vi "createState.vi"(8 "error in (no error)":errorcluster, 10 "State:":T1, 11 "StateFactory in":refnum<class "StateFactory.lvclass">) -> (0 "error out":errorcluster, 2 "State.lvclass":refnum<class "State.lvclass">, 3 "StateFactory out":refnum<class "StateFactory.lvclass">)   [LabVIEW 2013, in "StateFactory.lvclass"]
uses:
  StateFactory.lvclass
  Typedefs/StateSelector.ctl
  State/State.lvclass
  States/DataOnDemandState/DataOnDemandState.lvclass
  States/DataStreamingState/DataStreamingState.lvclass
  States/FaultState/FaultState.lvclass
  States/OffState/OffState.lvclass
  States/StandbyState/StandbyState.lvclass
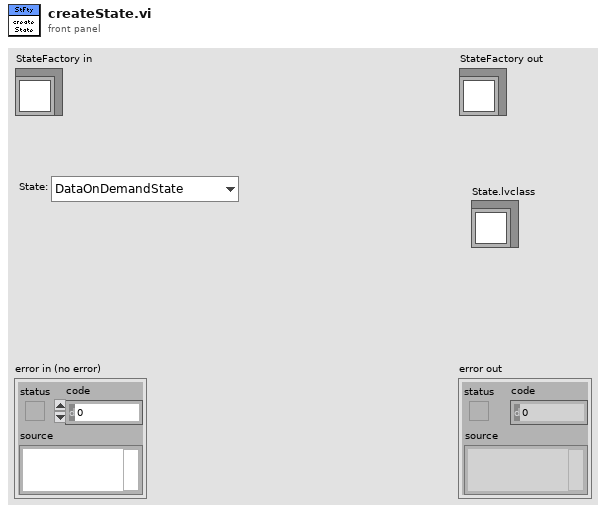
[diagram p1: front panel]
types:
  T1 = typedef "StateSelector.ctl" = enum16{"DataOnDemandState", "DataStreamingState", "FaultState", "OffState", "StandbyState"}
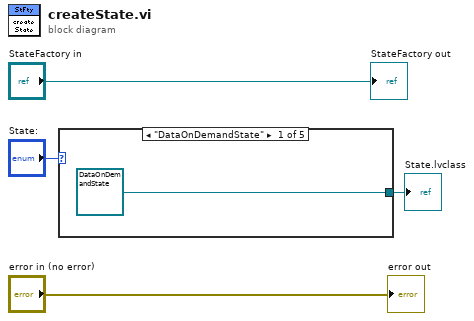
[diagram p0: block diagram]
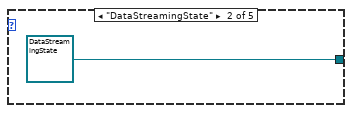
[diagram p2: hidden frame]
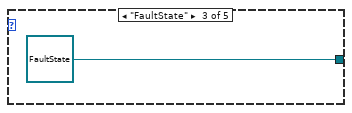
[diagram p3: hidden frame]
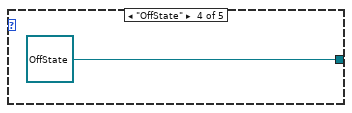
[diagram p4: hidden frame]
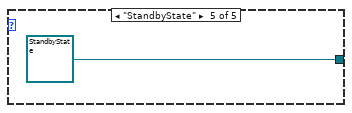
[diagram p5: hidden frame]
diagram:
  n1 = case shown="\"DataOnDemandState\"" "State:" {
    tunnel: [refnum<class "DataOnDemandState.lvclass"> refnum ("DataOnDemandState.lvclass") refnum<class "DataStreamingState.lvclass"> refnum ("DataStreamingState.lvclass") refnum<class "FaultState.lvclass"> refnum ("FaultState.lvclass") refnum<class "OffState.lvclass"> refnum ("ShutdownState.lvclass") refnum<class "StandbyState.lvclass"> refnum ("StandbyState.lvclass")] -> w1
    frame "DataOnDemandState" {
    }
    frame "DataStreamingState" {
    }
    frame "FaultState" {
    }
    frame "OffState" {
    }
    frame "StandbyState" {
    }
  }
  "State.lvclass" <- w1
  "error out" <- "error in (no error)"
  "StateFactory out" <- "StateFactory in"
